vi "FileMan Open File.vi"(7 "run minimized (F)":bool, 8 "error in (no error)":errorcluster, 9 "default directory (empty path)":path, 10 "command line parameters (\"\")":string, 11 "path to file (empty path)":path) -> (0 "error out":errorcluster)   [LabVIEW 2020, in "MacroAssert.lvlib" / "Winevent.lvlib"]
doc: "This VI will open a file whose extension is associated with an application, as available in Windows' File Manager, just as if you double-clicked on the file in File Manager. For example, files with the .wri extension are usually associated with the Windows application Write (write.exe). A file with the extension .wri will then be opened by Microsoft Write.\n\nAttempting to open files whose extensions are not associated with an application in the File Manager will result in an error."
uses:
  Winevent.lvlib
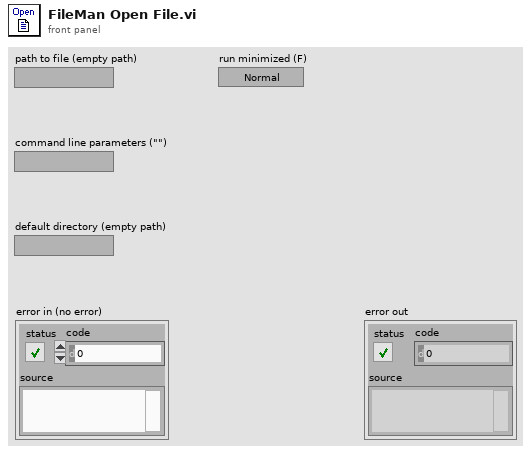
[diagram p1: front panel]
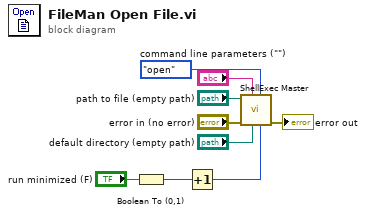
[diagram p0: block diagram]
diagram:
  n1 = Boolean To (0,1)(Boolean="run minimized (F)") -> (0, 1=w3:i16)
  n2 = Increment(x=w3) -> (x+1=w5:i16)
  n3 = call "ShellExec Master.vi"("show"=w5, "operation"=enum16{"open", "print"}."open", "default directory"="default directory (empty path)", "command line parameters"="command line parameters (\"\")", "error in (no error)"="error in (no error)", "path to file"="path to file (empty path)") -> ("error out"=→"error out":errorcluster)  [unwired: 5 in]
